vi "m1m3_getEvent_ForceActuatorState.vi"(8 "error in (no error)":errorcluster, 11 "logevent_ForceActuatorState_Ctl":T1) -> (0 "error out":errorcluster, 2 "function return":i32, 3 "logevent_ForceActuatorState_Ctl out":T1)   [LabVIEW 2016, in "SALLV_m1m3.lvlib"]
doc: "int m1m3_shm_getEvent_ForceActuatorStateLV(m1m3_logevent_ForceActuatorStateLV *logevent_ForceActuatorState_Ctl );"
uses:
  SALLV_m1m3.lvlib
  DataTypes/logevent_ForceActuatorState.ctl
  SALLV_m1m3.so
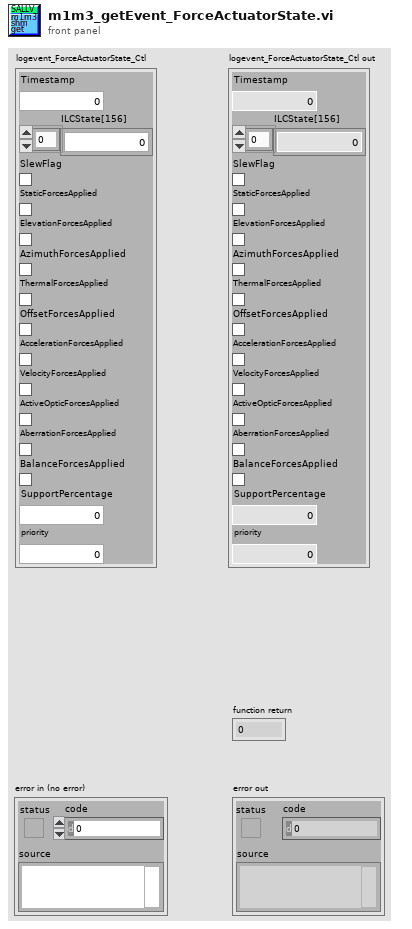
[diagram p1: front panel]
types:
  T1 = typedef "SALLV_m1m3.lvlib/logevent_ForceActuatorState.ctl" = cluster{"Timestamp":dbl, "ILCState[156]":i16[], "SlewFlag":bool, "StaticForcesApplied":bool, "ElevationForcesApplied":bool, "AzimuthForcesApplied":bool, "ThermalForcesApplied":bool, "OffsetForcesApplied":bool, "AccelerationForcesApplied":bool, "VelocityForcesApplied":bool, "ActiveOpticForcesApplied":bool, "AberrationForcesApplied":bool, "BalanceForcesApplied":bool, "SupportPercentage":sgl, "priority":i32}
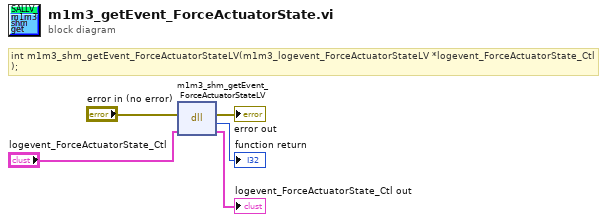
[diagram p0: block diagram]
diagram:
  # "int m1m3_shm_getEvent_ForceActuatorStateLV(m1m3_logevent_ForceActuatorStateLV *logevent_ForceActuatorState_Ctl );"
  n1 = dll-call lib="opt/CODE/SALLV_m1m3/SALLV_m1m3.*" fn="m1m3_shm_getEvent_ForceActuatorStateLV"(error in="error in (no error)", "logevent_ForceActuatorState_Ctl"="logevent_ForceActuatorState_Ctl") -> (error out=→"error out":errorcluster, →"function return":i32, "logevent_ForceActuatorState_Ctl"=→"logevent_ForceActuatorState_Ctl out":T1)  [unwired: 2 in, 1 out]
